vi "Limit Test Result.vi"(8 "error in (no error)":errorcluster, 9 "clear limit test (yes:T)":bool=TRUE, 10 "limit test function (1:one)":u16(ring)=1 items=["One"=1, "Two"=2], 11 "VISA resource name":refnum<visa-resource-name>) -> (0 "error out":errorcluster, 1 "result (pass :F)":bool, 3 "VISA resource name out":refnum<visa-resource-name>)   [LabVIEW 2016, in "Agilent 4263X.lvlib"]
doc: "This VI queries the limit test result fo the specified limit test function."
uses:
  <instrlib>/Agilent 4263X/Agilent 4263X.lvlib
panel:
  # "yes\nno"
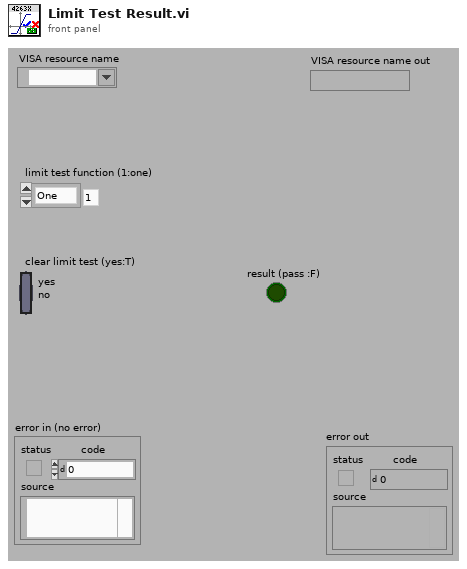
[diagram p1: front panel]
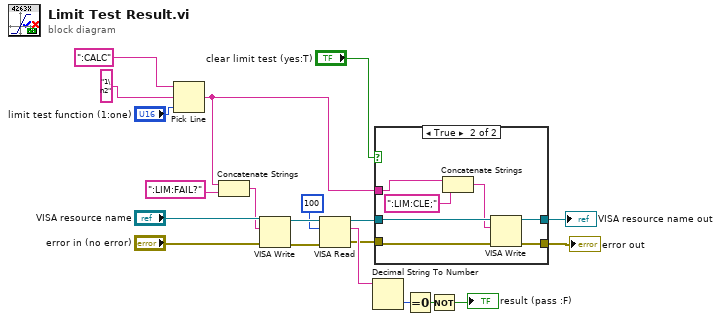
[diagram p0: block diagram]
diagram:
  n1 = Pick Line(string ("")=":CALC", multi-line string="1\n2", line index="limit test function (1:one)") -> (output string=w4:string)
  n2 = Concatenate Strings(w4, ":LIM:FAIL?") -> (w6:string)
  n3 = VISA Write(VISA resource name="VISA resource name", write buffer=w6, error in (no error)="error in (no error)") -> (VISA resource name out=w16:refnum<visa-resource-name>, error out=w15:errorcluster)  [unwired: 1 out]
  n4 = VISA Read(VISA resource name=w16, byte count=100, error in (no error)=w15) -> (VISA resource name out=w8:refnum<visa-resource-name>, read buffer=w13:string, error out=w7:errorcluster)  [unwired: 1 out]
  n5 = Decimal String To Number(string=w13) -> (number=w12:i32)  [unwired: 2 in, 1 out]
  n6 = case shown="True" "clear limit test (yes:T)" {
    tunnel: w8 -> [w22 w29]
    tunnel: w7 -> [w21 w28]
    tunnel: w4 -> [_ w27]
    tunnel: [w21 w24] -> w3
    tunnel: [w22 w23] -> w2
    frame False {
    }
    frame True {
      n7 = Concatenate Strings(w27, ":LIM:CLE;") -> (w26:string)
      n8 = VISA Write(VISA resource name=w29, write buffer=w26, error in (no error)=w28) -> (VISA resource name out=w23:refnum<visa-resource-name>, error out=w24:errorcluster)  [unwired: 1 out]
    }
  }
  "error out" <- w3
  "VISA resource name out" <- w2
  n9 = Equal To 0?(x=w12) -> (x = 0?=w11:bool)
  n10 = Not(x=w11) -> (.not. x?=→"result (pass :F)":bool)
